vi "Get Server gRPC UEs.vi"(11 "OOP Server in":refnum<class "OOP Server.lvclass">) -> (2 "Server gRPC UEs":T1, 3 "OOP Server out":refnum<class "OOP Server.lvclass">)   [LabVIEW 2019, in "OOP Server.lvclass"]
uses:
  OOP Server.lvclass
  gRPC interface/Server API/typeDefs/grpcId.ctl
  gRPC interface/gprc-lvsupport.lvlib
  gRPC interface/Server API/typeDefs/gRPCId Cluster.ctl
  gRPC interface/Server API/typeDefs/gRPCId Cluster UE.ctl
  typeDefs/Server gRPC UEs.ctl
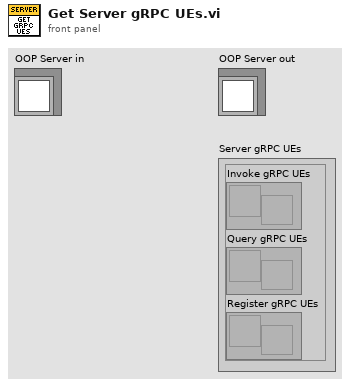
[diagram p1: front panel]
types:
  T1 = typedef "OOP Server.lvclass/Server gRPC UEs.ctl" = cluster{"Invoke gRPC UEs":T2, "Query gRPC UEs":T2, "Register gRPC UEs":T2}
  T2 = typedef "gprc-lvsupport.lvlib/gRPCId Cluster UE.ctl" = refnum<user-event>
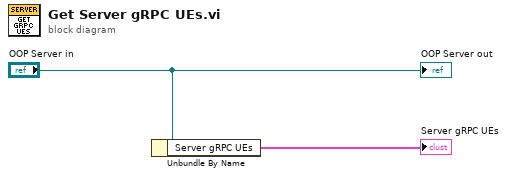
[diagram p0: block diagram]
diagram:
  n1 = Unbundle By Name("OOP Server in") -> ("Server gRPC UEs"=→"Server gRPC UEs":T1)
  "OOP Server out" <- "OOP Server in"
